vi "Get_Limits_V3.vi"(8 "Error In":errorcluster, 9 "Section":string, 10 "OutPutValue":u16(ring) items=["Numeric", "String"], 11 "FilePath":path) -> (0 "Error Out":errorcluster, 1 "ValueStr":string[](array[string]), 2 "ValueNum":dbl[](array[numeric]), 3 "Test Names":string[](array[string]), 4 "Boolean":bool, 5 "Test Limits":i32)   [LabVIEW 2022 SP3]
uses:
  <vilib>/Utility/config.llb/Read Key (String).vi
  <vilib>/Utility/config.llb/Read Key (Double).vi
  <vilib>/Utility/config.llb/NI_LVConfig.lvlib
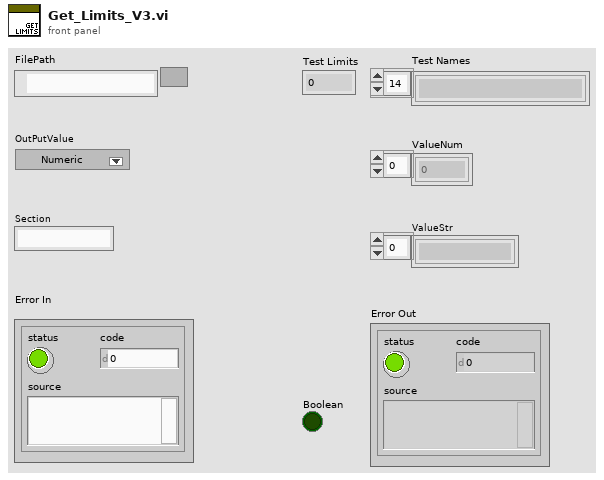
[diagram p1: front panel]
types:
  T1 = typedef "NI_LVConfig.lvlib/Config Data RefNum.ctl" = refnum<k1>
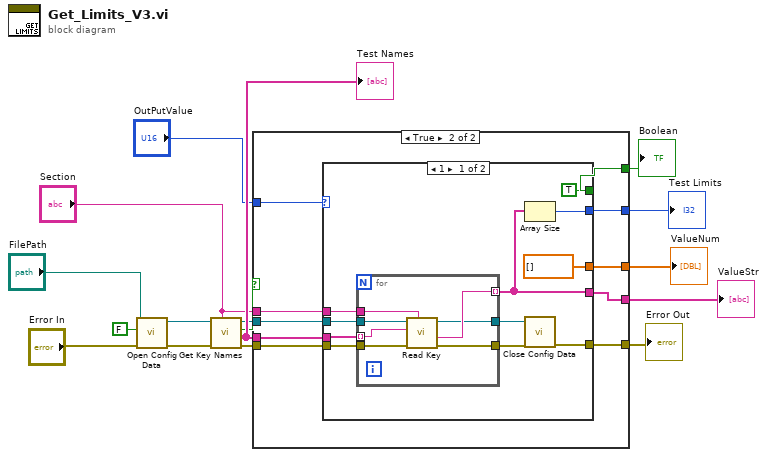
[diagram p0: block diagram]
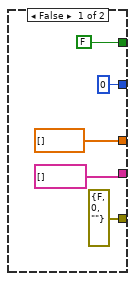
[diagram p2: hidden frame]
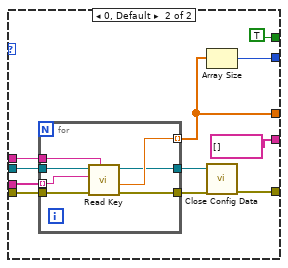
[diagram p3: hidden frame]
diagram:
  n1 = call <vilib>:"Open Config Data.vi"("error in (no error)"="Error In", "create file if necessary (T)"=FALSE, "configuration file path"="FilePath") -> ("error out"=w16:errorcluster, "refnum"=w15:T1)  [unwired: 6 in, 1 out]
  n2 = call <vilib>:"Get Key Names.vi"("section"="Section", "error in (no error)"=w16, "refnum"=w15) -> ("error out"=w14:errorcluster, "key names"=w13:string[], "section exists?"=w7:bool, "refnum out"=w12:T1)  [unwired: 5 in]
  "Test Names" <- w13
  n3 = case shown="True" w7 {
    tunnel: w14 -> [_ w31]
    tunnel: w13 -> [_ w30]
    tunnel: w12 -> [_ w29]
    tunnel: "Section" -> [_ w28]
    tunnel: [errorcluster {"status"=FALSE, "code"=0, "source"=""} ("error out") w27] -> w6
    tunnel: [0 w24] -> w5
    tunnel: [dbl[] [] w26] -> w4
    tunnel: [FALSE w25] -> w3
    tunnel: [string[] [] w23] -> w2
    tunnel: "OutPutValue" -> [_ w22]
    frame False {
    }
    frame True {
      n4 = case shown="1" w22 {
        tunnel: w31 -> [w37 w60]
        tunnel: w30 -> [w38 w59]
        tunnel: w29 -> [w39 w58]
        tunnel: w28 -> [w40 w57]
        tunnel: [w34 w54] -> w27
        tunnel: [w36 w53] -> w24
        tunnel: [dbl[] [] w52] -> w26
        tunnel: [TRUE TRUE] -> w25
        tunnel: [w33 string[] []] -> w23
        frame 1 {
          n5 = for {
            tunnel: w38 -> [w48] mode=indexing
            tunnel: w37 -> [w49]
            tunnel: w39 -> [w47]
            tunnel: w40 -> [w46]
            tunnel: [w45] -> w33 mode=indexing
            tunnel: [w44] -> w42
            tunnel: [w43] -> w41
            n6 = call-poly <vilib>:"Read Key.vi"("section"=w46, "error in (no error)"=w49, "key"=w48, "refnum"=w47) -> ("error out"=w44:errorcluster, "value"=w45:string, "refnum out"=w43:T1)  [unwired: 4 in, 1 out]
          }
          n7 = Array Size(array=w33) -> (size(s)=w36:i32)
          n8 = call <vilib>:"Close Config Data.vi"("error in (no error)"=w42, "refnum"=w41) -> ("error out"=w34:errorcluster)  [unwired: 8 in, 1 out]
        }
        frame 0, Default {
          n9 = for {
            tunnel: w59 -> [w66] mode=indexing
            tunnel: w60 -> [w67]
            tunnel: w58 -> [w65]
            tunnel: w57 -> [w64]
            tunnel: [w63] -> w52 mode=indexing
            tunnel: [w62] -> w56
            tunnel: [w61] -> w55
            n10 = call-poly <vilib>:"Read Key.vi"("section"=w64, "error in (no error)"=w67, "key"=w66, "refnum"=w65) -> ("error out"=w62:errorcluster, "value"=w63:dbl, "refnum out"=w61:T1)  [unwired: 4 in, 1 out]
          }
          n11 = Array Size(array=w52) -> (size(s)=w53:i32)
          n12 = call <vilib>:"Close Config Data.vi"("error in (no error)"=w56, "refnum"=w55) -> ("error out"=w54:errorcluster)  [unwired: 8 in, 1 out]
        }
      }
    }
  }
  "Error Out" <- w6
  "Test Limits" <- w5
  "ValueNum" <- w4
  "Boolean" <- w3
  "ValueStr" <- w2
